vi "MicronService.vi"() -> ()   [LabVIEW 2019]
doc: "TCP Server Example. After running this VI, run the Client Write or Write Read Example."
uses:
  <vilib>/SLL Toolkit/SLL Easy TCP/SLL Easy API via TCP.lvclass
  <vilib>/Utility/error.llb/DialogType.ctl
  <vilib>/SLL Toolkit/SLL Queued State Machine/Queue Driver/Create Queue.vi
  <vilib>/SLL Toolkit/SLL Queued State Machine/Queue Driver/Enqueue an Item to Queue.vi
  <vilib>/SLL Toolkit/SLL Queued State Machine/Queue Driver/Dequeue Queue.vi
  <vilib>/SLL Toolkit/SLL Easy TCP/_SubVIs/TCP Initialize Server - Local.vi
  <vilib>/SLL Toolkit/SLL Queued State Machine/Queue Driver/Enqueue N Items.vi
  <vilib>/SLL Toolkit/SLL Queued State Machine/Queue Driver/Flush Queue.vi
  <vilib>/SLL Toolkit/SLL Queued State Machine/Queue Driver/Release Queue.vi
  <vilib>/SLL Toolkit/SLL Queued State Machine/SLL QSM.lvlib
  <vilib>/SLL Toolkit/SLL String/SLL String.lvlib
panel:
  out "Service Name":string
  out "Last Command Time":string
  out "error out":errorcluster
  out "Last Command":string
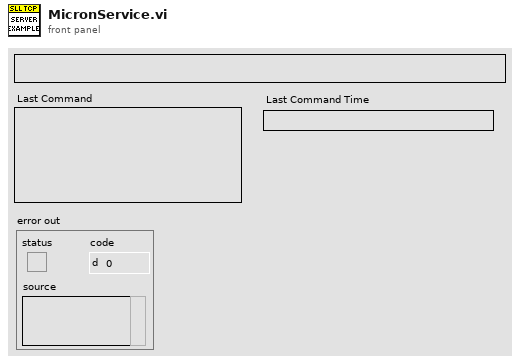
[diagram p1: front panel]
types:
  T1 = enum32{"Invalid", "Standard", "Closed", "Hidden", "Minimized", "Maximized"}
  T2 = cluster{"Flags":cluster{"Source Code?":bool}, "SLL TCP":refnum<class "SLL Easy API via TCP.lvclass">, "ServiceName":string, "UI":cluster{"Hide?":bool}}
  T3 = typedef "DialogType.ctl" = u16
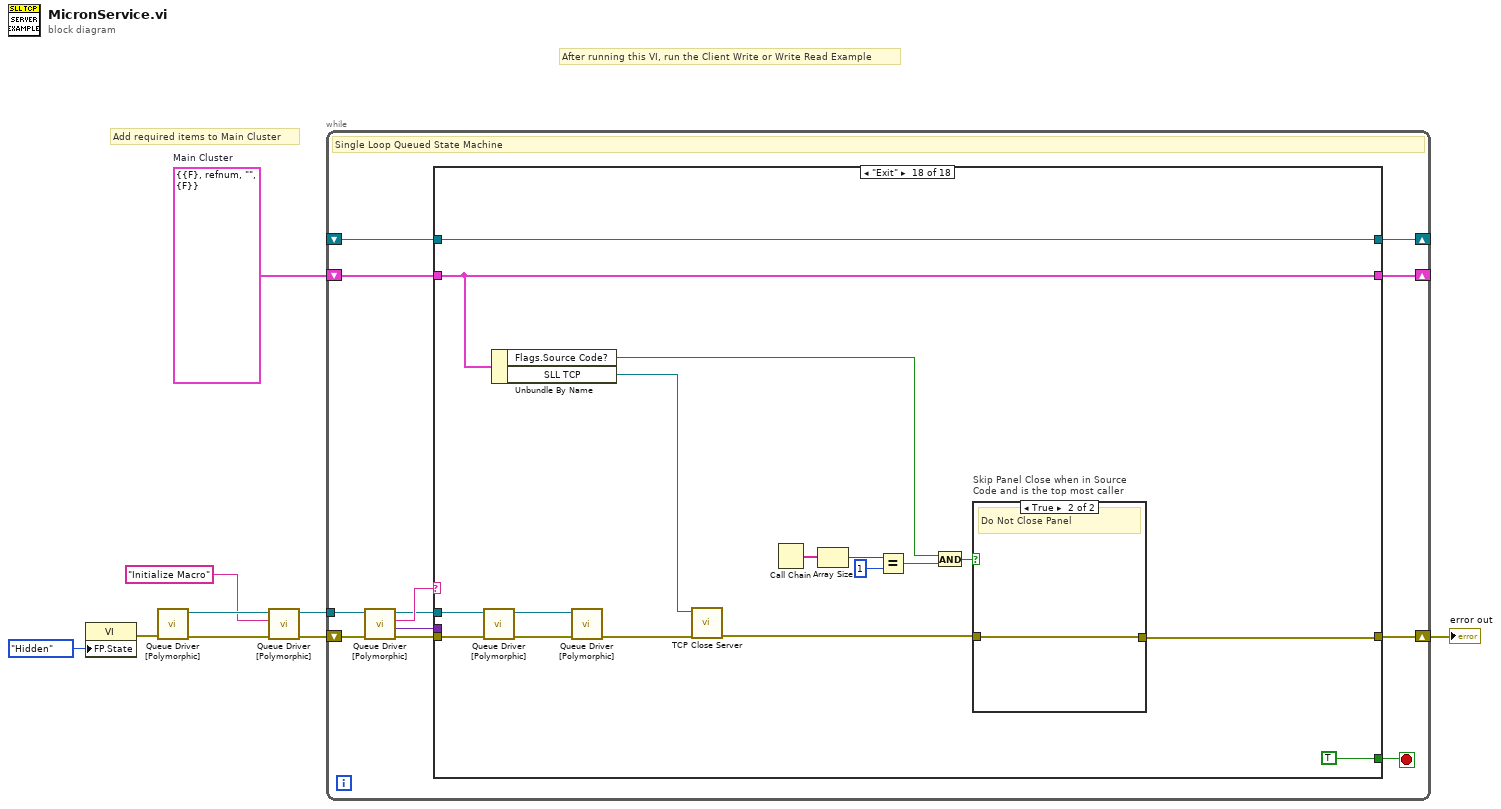
[diagram p0: block diagram]
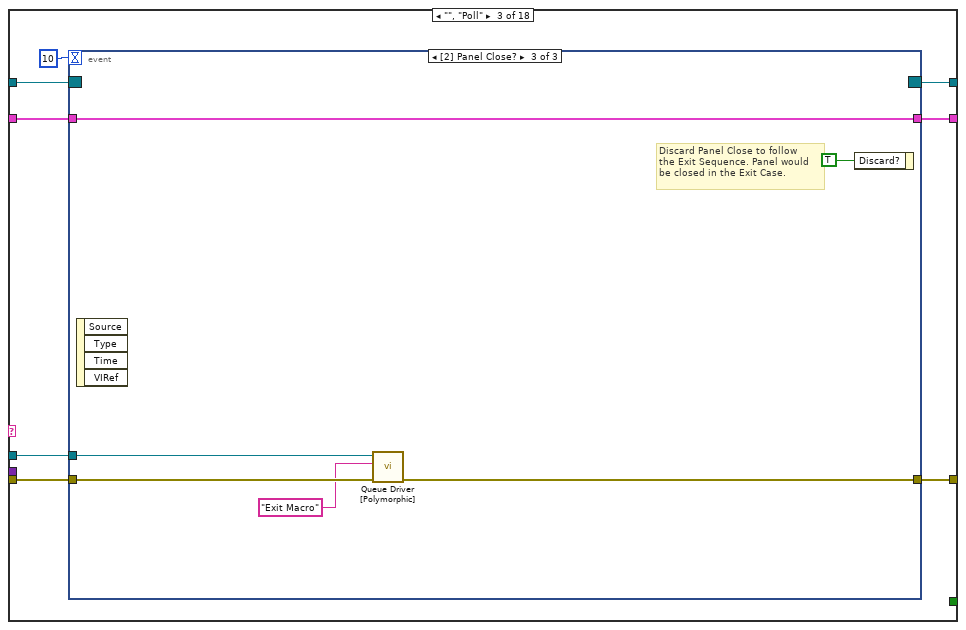
[diagram p4: hidden frame]
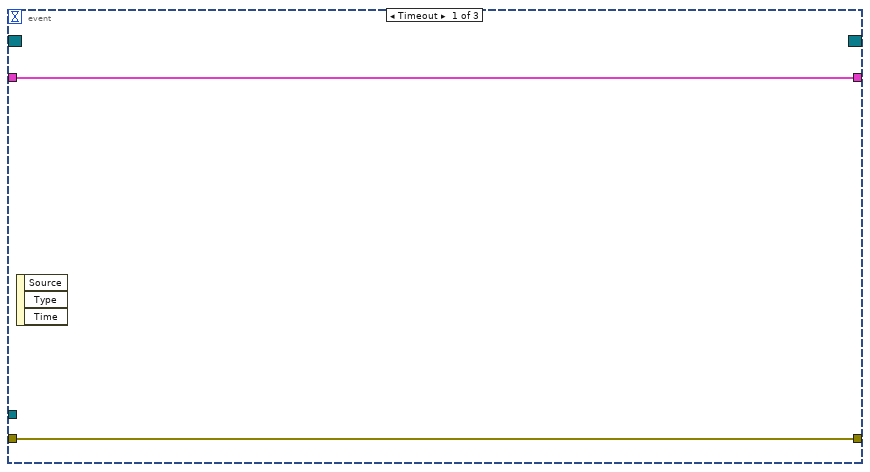
[diagram p5: hidden frame]
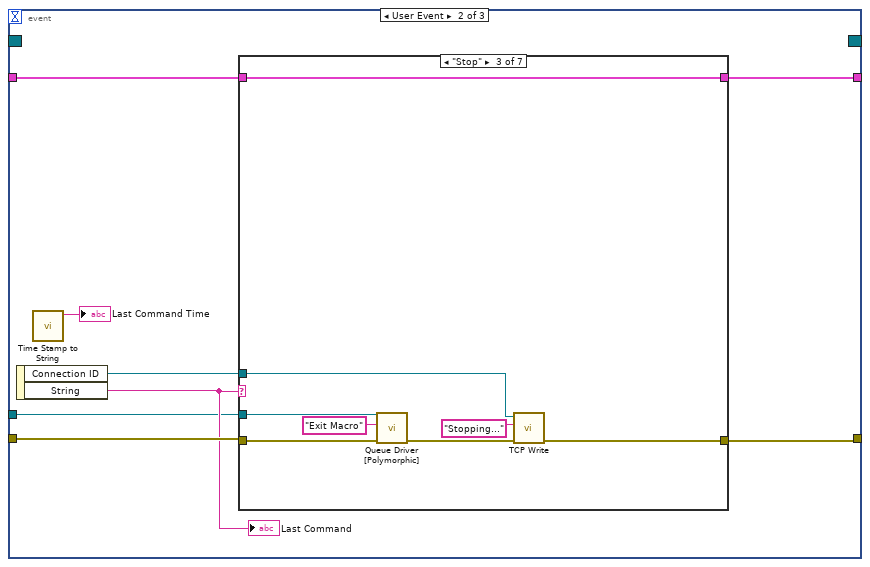
[diagram p6: hidden frame]
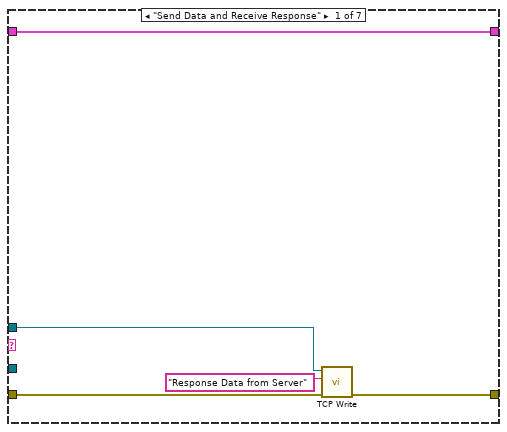
[diagram p7: hidden frame]
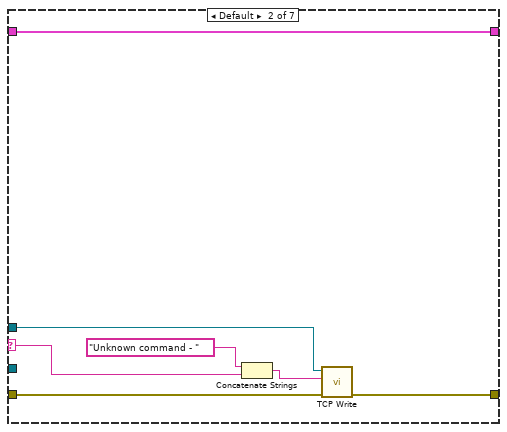
[diagram p8: hidden frame]
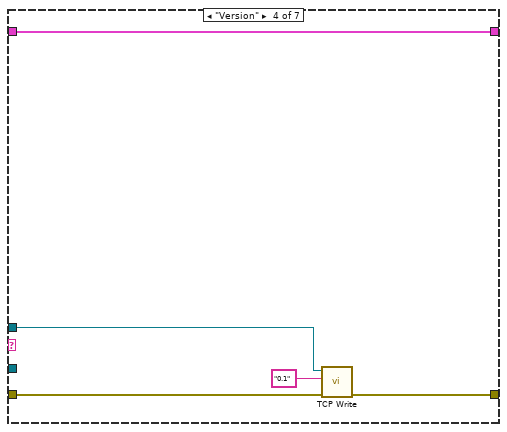
[diagram p9: hidden frame]
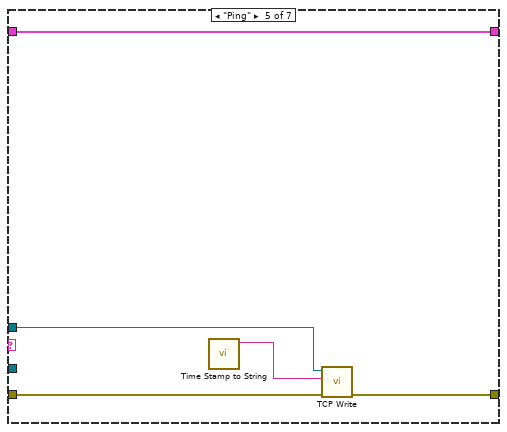
[diagram p10: hidden frame]
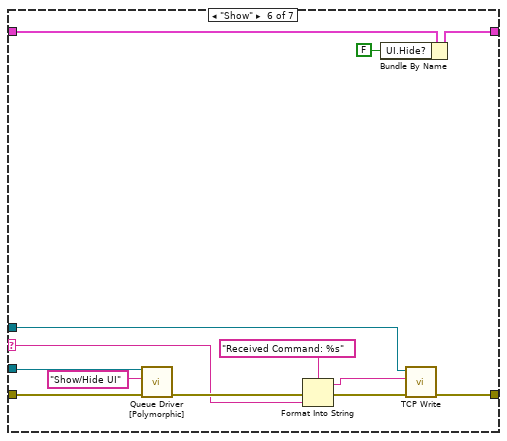
[diagram p11: hidden frame]
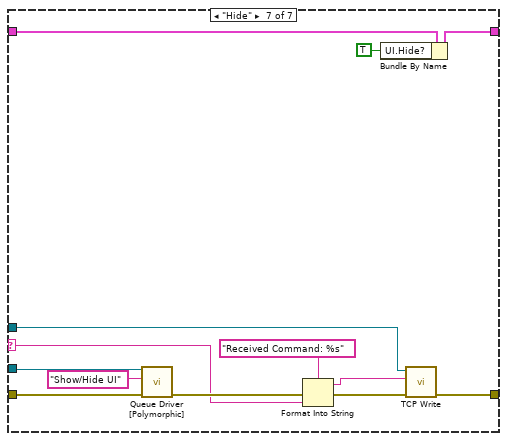
[diagram p12: hidden frame]
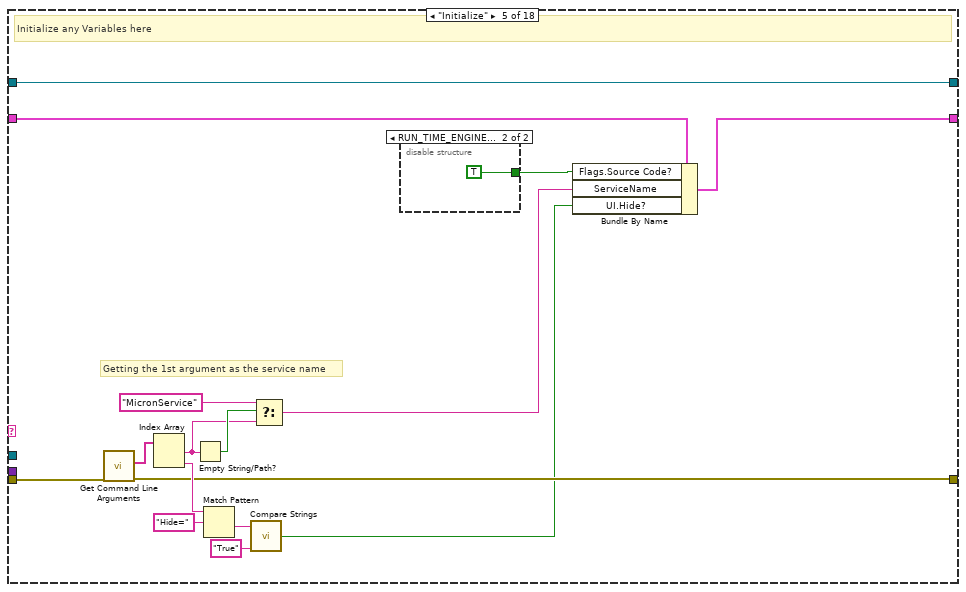
[diagram p14: hidden frame]
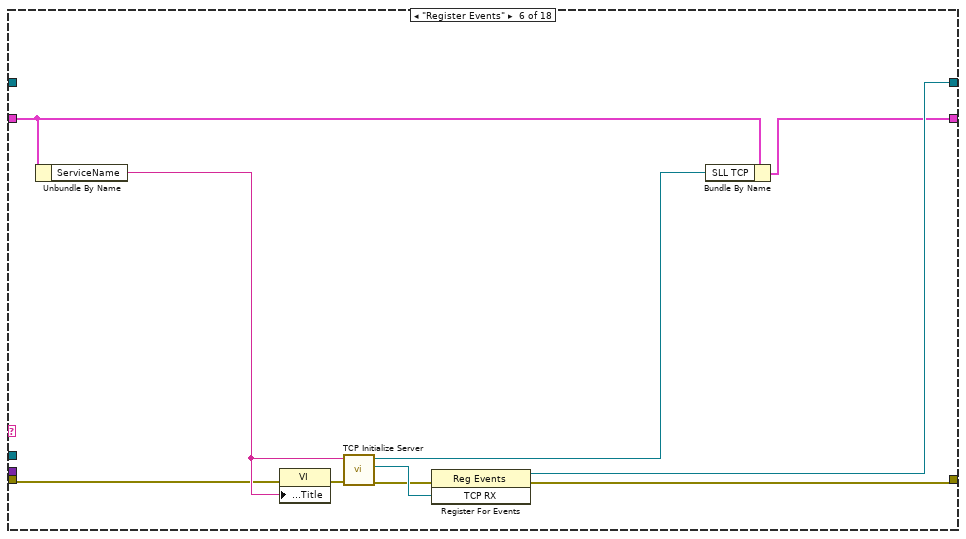
[diagram p16: hidden frame]
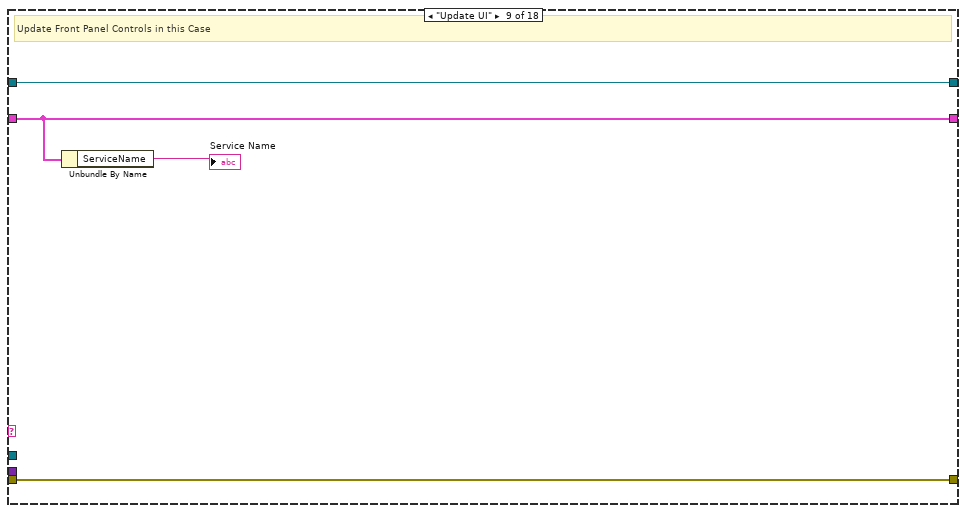
[diagram p19: hidden frame]
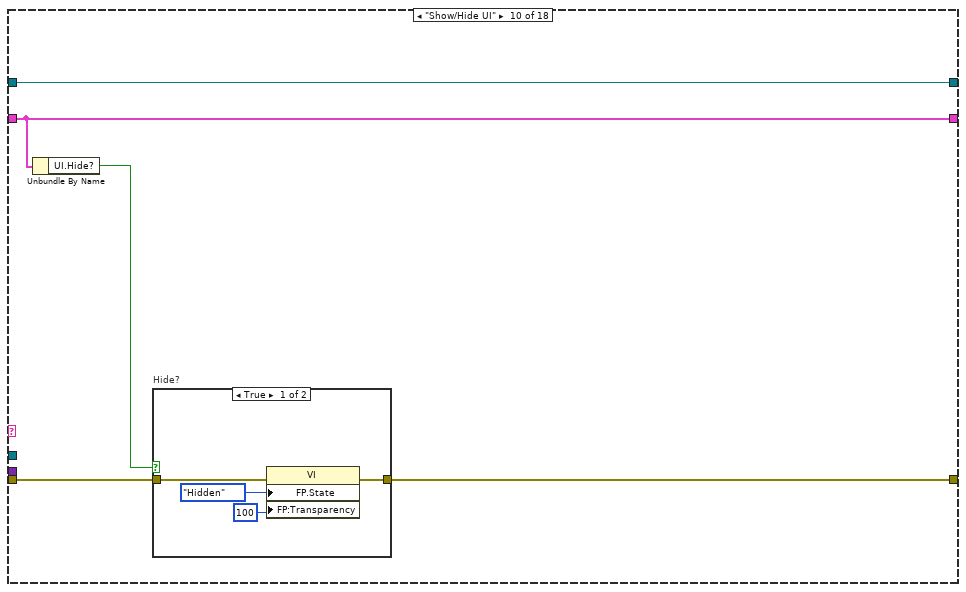
[diagram p20: hidden frame]
diagram:
  w6 = T2 {"Flags"={"Source Code?"=FALSE}, "SLL TCP"=refnum, "ServiceName"="", "UI"={"Hide?"=FALSE}}  # Main Cluster
  # "Add required items to Main Cluster"
  # "After running this VI, run the Client Write or Write Read Example"
  n1 = property class="VI"("FP.State"=T1."Hidden" ("Front Panel Window:State")) -> (error out=w2:errorcluster)  [unwired: 2 in, 1 out]
  n2 = call-poly <vilib>:"Queue Driver [Polymorphic].vi"("Error In"=w2) -> ("Error Out"=w4:errorcluster, "Queue Ref"=w8:refnum<queue>)  [unwired: 9 in]
  n3 = call-poly <vilib>:"Queue Driver [Polymorphic].vi"("Error In"=w4, "Item to Add"="Initialize Macro", "Queue Ref In"=w8) -> ("Error Out"=w5:errorcluster, "Queue Ref Out"=w9:refnum<queue>)  [unwired: 7 in]
  n4 = while "SLL Queued State Machine" {
    shift-right: [w19] -> w3
    shift-left: w5 -> [w21]
    shift-right: [w17] -> _
    shift-left: _ -> [w16]
    shift-right: [w15] -> _
    shift-left: w6 -> [w14]
    tunnel: w9 -> [w12]
    stop <- w18 stop-if-true
    # "Single Loop Queued State Machine"
    n5 = call-poly <vilib>:"Queue Driver [Polymorphic].vi"("Error In"=w21, "Queue Ref In"=w12) -> ("Error Out"=w20:errorcluster, "Data"=w10:variant, "Dequeue"=w13:string, "Queue Ref Out"=w11:refnum<queue>)  [unwired: 6 in]
    n6 = case "QSM Case Structure" shown="\"Exit\"" w13 {
      selector: w13 -> [_ _ _ _ _ _ _ _ _ _ _ _ _ _ w181 _ _ _]
      tunnel: w20 -> [w24 w27 w33 w110 w118 w128 w140 w143 w144 w151 w163 w167 w175 w180 w184 w196 w199 w214]
      tunnel: [w24 w27 w34 w110 w114 w134 w140 w143 w144 w150 w163 w166 w174 w180 w187 w194 w199 w211] -> w19
      tunnel: [_ _ _ _ _ _ _ _ _ _ _ _ _ _ _ _ _ TRUE] -> w18
      tunnel: [w23 w26 w32 w109 w126 w133 w139 w142 w147 w152 w162 w169 w177 w179 w190 w193 w198 w213] -> w17
      tunnel: w16 -> [w23 w26 w31 w109 w126 _ w139 w142 w147 w152 w162 w169 w177 w179 w190 w193 w198 w213]
      tunnel: [w22 w25 w29 w108 w123 w132 w138 w141 w146 w149 w161 w168 w171 w178 w189 w192 w197 w212] -> w15
      tunnel: w14 -> [w22 w25 w30 w108 w124 w130 w138 w141 w146 w149 w161 w168 w176 w178 w189 w192 w197 w212]
      tunnel: w11 -> [_ _ w28 _ _ _ _ _ _ _ _ w165 w172 _ _ _ _ w204]
      tunnel: w10 -> [_ _ _ _ _ _ _ _ _ _ _ _ _ _ _ _ _ _]
      frame "/--------------- Read Me -----------------/" {
        # "General Purpose Queue Based State Machine for Any Use Case (main application, module, pop up message etc)\n\nAdvantages:\n1. Lean Project Code Base (dependencies are in vilib).\n2. This template can be safely used in multiple parallel running modules without any issues.\n3. This template can also be safely used even in cases where the VI is configured to be a clone, where multiple \ninstances of the VI could be executing concurrently.\n\nHow to Use:\n1. Add necessary items to the Main Cluster.\n2. Use the Polymorphic Queue Driver for doing any queue operations. \n3. Add any required user events in the \"Register Events\" case. Ignore if not needed.\n4. Use \"Macros\" section for defining any list of state calls, which could be used in multiple places. \nEx: Initialize Macro, might be needed if we need to any reinitialization."
      }
      frame "/------------------ Poll -------------------/" {
      }
      frame "", "Poll" {
        n7 = event shown="[2] Panel Close?" {
          selector: w31 -> [_ _ _]
          dyn-events: [_ _ _] -> w32
          timeout: 10 -> [_ _ _]
          tunnel: [w37 w43 w106] -> w34
          tunnel: w33 -> [w37 w44 w107]
          tunnel: w30 -> [w36 w39 w105]
          tunnel: [w36 w38 w105] -> w29
          tunnel: w28 -> [_ w40 w103]
          event Timeout {
            n8 = event-data() -> ()  [unwired: 1 in, 3 out]
          }
          event User Event {
            n9 = event-data() -> ("Connection ID"=w41:refnum<k5>, "String"=w42:string)  [unwired: 1 in]
            "Last Command" <- w42
            n10 = call <vilib>:"Time Stamp to String.vi"() -> ("Output String"=→"Last Command Time":string)  [unwired: 11 in]
            n11 = case shown="\"Stop\"" w42 {
              selector: w42 -> [_ w53 _ _ _ w77 w90]
              tunnel: w41 -> [w50 w57 w65 w70 w75 w88 w101]
              tunnel: w44 -> [w48 w56 w62 w68 w74 w85 w98]
              tunnel: [w47 w55 w59 w67 w73 w87 w100] -> w43
              tunnel: w40 -> [_ _ w61 _ _ w83 w96]
              tunnel: w39 -> [w46 w51 w58 w66 w71 w82 w95]
              tunnel: [w46 w51 w58 w66 w71 w81 w94] -> w38
              frame "Send Data and Receive Response" {
                n12 = call <vilib>:"TCP Write.vi"("error in (no error)"=w48, "Write Data"="Response Data from Server", "connection ID In"=w50) -> ("error out"=w47:errorcluster)  [unwired: 7 in, 1 out]
              }
              frame Default {
                n13 = Concatenate Strings("Unknown command - " ("Write Data"), w53) -> (w52:string)
                n14 = call <vilib>:"TCP Write.vi"("error in (no error)"=w56, "Write Data"=w52, "connection ID In"=w57) -> ("error out"=w55:errorcluster)  [unwired: 7 in, 1 out]
              }
              frame "Stop" {
                n15 = call-poly <vilib>:"Queue Driver [Polymorphic].vi"("Error In"=w62, "Item to Add"="Exit Macro" ("Enqueue"), "Queue Ref In"=w61) -> ("Error Out"=w60:errorcluster)  [unwired: 7 in, 1 out]
                n16 = call <vilib>:"TCP Write.vi"("error in (no error)"=w60, "Write Data"="Stopping...", "connection ID In"=w65) -> ("error out"=w59:errorcluster)  [unwired: 7 in, 1 out]
              }
              frame "Version" {
                n17 = call <vilib>:"TCP Write.vi"("error in (no error)"=w68, "Write Data"="0.1", "connection ID In"=w70) -> ("error out"=w67:errorcluster)  [unwired: 7 in, 1 out]
              }
              frame "Ping" {
                n18 = call <vilib>:"Time Stamp to String.vi"() -> ("Output String"=w72:string)  [unwired: 11 in]
                n19 = call <vilib>:"TCP Write.vi"("error in (no error)"=w74, "Write Data"=w72, "connection ID In"=w75) -> ("error out"=w73:errorcluster)  [unwired: 7 in, 1 out]
              }
              frame "Show" {
                n20 = call-poly <vilib>:"Queue Driver [Polymorphic].vi"("Error In"=w85, "Item to Add"="Show/Hide UI" ("Enqueue"), "Queue Ref In"=w83) -> ("Error Out"=w84:errorcluster)  [unwired: 7 in, 1 out]
                n21 = Format Into String(format string="Received Command: %s", error in=w84, w77) -> (resulting string=w76:string, error out=w79:errorcluster)  [unwired: 1 in]
                n22 = Bundle By Name(cluster=w82, "UI.Hide?"=FALSE) -> (w81:T2)
                n23 = call <vilib>:"TCP Write.vi"("error in (no error)"=w79, "Write Data"=w76, "connection ID In"=w88) -> ("error out"=w87:errorcluster)  [unwired: 7 in, 1 out]
              }
              frame "Hide" {
                n24 = call-poly <vilib>:"Queue Driver [Polymorphic].vi"("Error In"=w98, "Item to Add"="Show/Hide UI" ("Enqueue"), "Queue Ref In"=w96) -> ("Error Out"=w97:errorcluster)  [unwired: 7 in, 1 out]
                n25 = Format Into String(format string="Received Command: %s", error in=w97, w90) -> (resulting string=w89:string, error out=w92:errorcluster)  [unwired: 1 in]
                n26 = Bundle By Name(cluster=w95, "UI.Hide?"=TRUE) -> (w94:T2)
                n27 = call <vilib>:"TCP Write.vi"("error in (no error)"=w92, "Write Data"=w89, "connection ID In"=w101) -> ("error out"=w100:errorcluster)  [unwired: 7 in, 1 out]
              }
            }
          }
          event Panel Close? {
            # "Discard Panel Close to follow\nthe Exit Sequence. Panel would\nbe closed in the Exit Case."
            n28 = event-data() -> ()  [unwired: 1 in, 4 out]
            n29 = call-poly <vilib>:"Queue Driver [Polymorphic].vi"("Error In"=w107, "Item to Add"="Exit Macro" ("Enqueue"), "Queue Ref In"=w103) -> ("Error Out"=w106:errorcluster)  [unwired: 7 in, 1 out]
            n30 = event-data("Discard?"=TRUE) -> ()  [unwired: 1 in, 1 out]
          }
        }
      }
      frame "/--------------- Initialize -----------------/" {
      }
      frame "Initialize" {
        # "Getting the 1st argument as the service name"
        # "Initialize any Variables here"
        n31 = call <vilib>:"Get Command Line Arguments.vi"("error in (no error)"=w118) -> ("error out"=w114:errorcluster, "arguments"=w122:string[])  [unwired: 8 in, 1 out]
        n32 = Index Array(array=w122) -> (element #1=w120:string, element #2=w116:string)  [unwired: 2 in]
        n33 = Empty String/Path?(string/path=w120) -> (empty?=w121:bool)
        n34 = Match Pattern(string=w116, regular expression="Hide=") -> (after substring=w113:string)  [unwired: 1 in, 3 out]
        n35 = call <vilib>:"Compare Strings.vi"("y"="True", "x"=w113) -> ("Equal?"=w111:bool)
        n36 = Select(t="MicronService", s=w121, f=w120) -> (s? t:f=w117:string)
        n37 = disable-structure shown="RUN_TIME_ENGINE==False" {
          disable-tunnel: [_ TRUE] -> w125
          frame condition #0 {
          }
          frame condition #1 (active) {
          }
        }
        n38 = Bundle By Name(cluster=w124, "Flags.Source Code?"=w125, "ServiceName"=w117, "UI.Hide?"=w111) -> (w123:T2)
      }
      frame "Register Events" {
        n39 = Unbundle By Name(w130) -> ("ServiceName"=w129:string)
        n40 = property class="VI"(error in=w128, "Front Panel.Title"=w129) -> (error out=w135:errorcluster)  [unwired: 1 in, 1 out]
        n41 = call-poly <vilib>:"TCP Initialize Server.vi"("error in (no error)"=w135, "Service Name"=w129) -> ("error out"=w136:errorcluster, "TCP RX"=w137:refnum<user-event>, "SLL Easy API via TCP out"=w131:refnum<class "SLL Easy API via TCP.lvclass">)  [unwired: 7 in]
        n42 = register-events(error in=w136, w137) -> (reference out=w133:refnum<event-registration>, error out=w134:errorcluster)  [unwired: 1 in]
        n43 = Bundle By Name(cluster=w130, "SLL TCP"=w131) -> (w132:T2)
      }
      frame "/---------- Custom Case Splitter ----------/" {
      }
      frame "/-------------- User Interface --------------/" {
        # "Duplicate this case to create additional case splitters for readability"
      }
      frame "Update UI" {
        # "Update Front Panel Controls in this Case"
        n44 = Unbundle By Name(w146) -> ("ServiceName"=→"Service Name":string)
      }
      frame "Show/Hide UI" {
        n45 = Unbundle By Name(w149) -> ("UI.Hide?"=w148:bool)
        n46 = case "Hide?" shown="True" w148 {
          tunnel: w151 -> [w154 w158]
          tunnel: [w153 w157] -> w150
          frame True {
            n47 = property class="VI"(error in=w154, "FP.State"=T1."Hidden" ("Front Panel Window:State"), "FP:Transparency"=u8 100 ("Front Panel Window:Transparency")) -> (error out=w153:errorcluster)  [unwired: 1 in, 1 out]
          }
          frame False {
            n48 = property class="VI"(error in=w158, "FP.State"=T1."Standard" ("Front Panel Window:State"), "FP:Transparency"=u8 0 ("Front Panel Window:Transparency")) -> (error out=w157:errorcluster)  [unwired: 1 in, 1 out]
          }
        }
      }
      frame "/----------------- Macros -----------------/" {
      }
      frame "Initialize Macro" {
        w164 = string[] ["Initialize", "Register Events", "Show/Hide UI", "Update UI"]  # Initialize Macro
        n49 = call-poly <vilib>:"Queue Driver [Polymorphic].vi"("Error In"=w167, "Enqueue N"=w164, "Queue Ref In"=w165) -> ("Error Out"=w166:errorcluster)  [unwired: 7 in, 1 out]
      }
      frame "Exit Macro" {
        n50 = call-poly <vilib>:"Queue Driver [Polymorphic].vi"("Error In"=w175, "Enqueue N"=string[] ["Show/Hide UI", "Exit"], "Queue Ref In"=w172) -> ("Error Out"=w174:errorcluster)  [unwired: 7 in, 1 out]
        n51 = Bundle By Name(cluster=w176, "UI.Hide?"=TRUE) -> (w171:T2)
      }
      frame "/-------------- Error Handler--------------/" {
      }
      frame Default {
        # "Undefined Case/Spelling Errors - Show Message to Developer"
        n52 = property class="VI"(error in=w184) -> (error out=w183:errorcluster, "Name"=w182:string)  [unwired: 1 in, 1 out]
        n53 = Format Into String(format string="\"%s\" in the VI - %s" ("message"), initial string="Undefined case - ", error in=w183, w181, w182) -> (resulting string=w185:string, error out=w187:errorcluster)
        n54 = One Button Dialog(message=w185) -> ()  [unwired: 1 in, 1 out]
      }
      frame "Error" {
        w191 = T3 2 items=["no dialog", "OK message", "continue or stop message", "OK message + warnings", "continue/stop + warnings"] ("type of dialog (OK msg:1)")
        # "Handle the Error"
        n55 = call <vilib>:"Simple Error Handler.vi"("type of dialog (OK msg:1)"=w191, "error in (no error)"=w196) -> ("error out"=w195:errorcluster)  [unwired: 3 in, 4 out]
        n56 = call <vilib>:"Clear Errors.vi"("error in (no error)"=w195) -> ("error out"=w194:errorcluster)  [unwired: 5 in, 1 out]
      }
      frame "/------------------- Exit --------------------/" {
      }
      frame "Exit" {
        n57 = call-poly <vilib>:"Queue Driver [Polymorphic].vi"("Error In"=w214, "Queue Ref In"=w204) -> ("Error Out"=w215:errorcluster, "Queue Ref Out"=w203:refnum<queue>)  [unwired: 7 in, 1 out]
        n58 = Unbundle By Name(w212) -> ("Flags.Source Code?"=w206:bool, "SLL TCP"=w201:refnum<class "SLL Easy API via TCP.lvclass">)
        n59 = call-poly <vilib>:"Queue Driver [Polymorphic].vi"("Error In"=w215, "Queue Ref In"=w203) -> ("Error Out"=w202:errorcluster)  [unwired: 9 in]
        n60 = call <vilib>:"TCP Close Server.vi"("error in (no error)"=w202, "SLL Easy API via TCP in"=w201) -> ("error out"=w200:errorcluster)  [unwired: 9 in]
        n61 = Call Chain() -> (call chain=w210:string[])
        n62 = Array Size(array=w210) -> (size(s)=w209:i32)
        n63 = Equal?(x=w209, y=1) -> (x = y?=w207:bool)
        n64 = And(x=w206, y=w207) -> (x .and. y?=w205:bool)
        n65 = case "Skip Panel Close when in Source\nCode and is the top most caller" shown="True" w205 {
          tunnel: w200 -> [w218 w220]
          tunnel: [w219 w220] -> w211
          frame False {
            # "Close Panel"
            n66 = invoke class="VI" method="FP.Close"() -> (error out=w217:errorcluster)  [unwired: 3 in, 2 out]
            n67 = Merge Errors(w218, w217) -> (w219:errorcluster)
          }
          frame True {
            # "Do Not Close Panel"
          }
        }
      }
    }
  }
  "error out" <- w3
